vi "Init Platform Plugins.vi"(8 "error in (no error)":errorcluster, 11 "GVIWebProcessorApp in":refnum<class "GVIWebProcessorApp.lvclass">) -> (0 "error out":errorcluster, 3 "GVIWebProcessorApp out":refnum<class "GVIWebProcessorApp.lvclass">)   [LabVIEW 2020, in "PicoG-Processor.lvlib" / "GVIWebProcessorApp.lvclass"]
uses:
  GVIWebProcessorApp.lvclass
  Builds/picoG/ppl/PicoG-Core.lvlibp/PicoG-Processor/PicoG-Core/PlatformPluginManager/PlatformPluginManager.lvclass
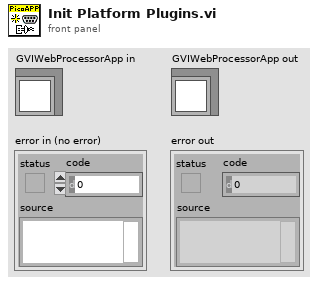
[diagram p1: front panel]
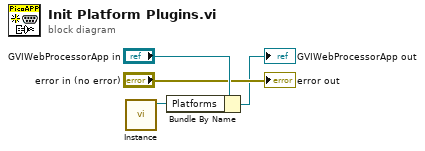
[diagram p0: block diagram]
diagram:
  n1 = call "Instance.vi"() -> ("Platform Manager"=w1:refnum<class "PlatformPluginManager.lvclass">)  [unwired: 10 in, 1 out]
  n2 = Bundle By Name(cluster="GVIWebProcessorApp in", "Platforms"=w1) -> (→"GVIWebProcessorApp out":refnum<class "GVIWebProcessorApp.lvclass">)
  "error out" <- "error in (no error)"
